vi "Pack for gRPC.vi"(8 "error in":errorcluster, 9 "configuration / results":enum16{"Configuration", "Results"}(ring), 10 "data value":variant, 11 "measurement customizations in":refnum<class "Measurement Plugin.lvclass">) -> (0 "error out":errorcluster, 2 "any":T1, 3 "measurement customizations out":refnum<class "Measurement Plugin.lvclass">)   [LabVIEW 2021, in "PWM Dimming.lvlib" / "Measurement Plugin.lvclass"]
uses:
  Measurement Plugin.lvclass
  Measurement Plugin.lvclass/Measurement Plugin.ctl
  Measurement Configuration.ctl
  PWM Dimming.lvlib
  Measurement Results.ctl
  a6012965-5700-4384-8228-972e71b6560c.vi
  2eca732d-dbaa-43bf-a7dd-ede2da65bc1b.vi
  <vilib>/Plug-In SDKs/Measurements/Measurement Plugin Service/Measurement Plugin Service.lvclass
  C:/Program Files/National Instruments/LabVIEW 2021/vi.lib/Plug-In SDKs/Measurements/Measurement Plugin Service/Measurement Plugin Service.lvclass
  <vilib>/gRPC/LabVIEW gRPC Library/Shared/Any.ctl
  <vilib>/gRPC/LabVIEW gRPC Library/grpc-lvsupport-release.lvlib
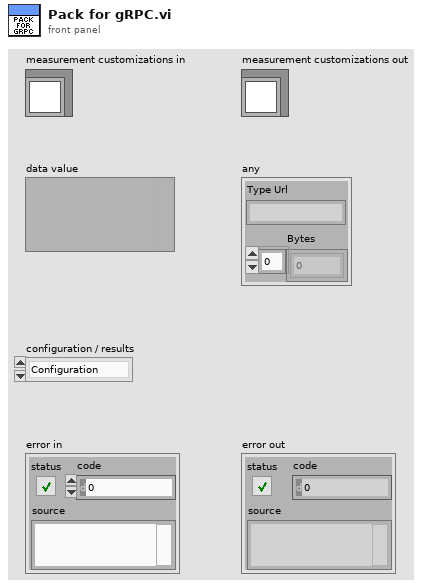
[diagram p1: front panel]
types:
  T1 = typedef "grpc-lvsupport-release.lvlib/Any.ctl" = cluster{"Type Url":string, "Bytes":u8[]}
  T2 = typedef "grpc-lvsupport-release.lvlib/grpcId.ctl" = u64
  T3 = typedef "PWM Dimming.lvlib/Measurement Configuration.ctl" = cluster{"DUT setup time":dbl, "Nominal output voltage":dbl, "Duty cycle single pulse/sweep pulse":bool, "PWM frequency":dbl, "Start duty cycle":dbl, "Stop duty cycle":dbl, "Number of sweep points":i32, "Duty cycle sweep type":string, "Duty cycle single point":dbl, "Number of pulse cycle":i32, "Source resource name":string, "Source sense":i32, "Source voltage level":dbl, "Source voltage level range":dbl, "Source transient response":i32, "Source voltage gain bandwidth":dbl, "Source voltage compensation frequency":dbl, "Source voltage pole-zero ratio":dbl, "Load resource name":string, "Load sense":i32, "Load pulse current level":dbl, "Load pulse bias current level":dbl, "Load sample rate":dbl, "Load voltage limit range":dbl, "Load transient response":i32, "Load current gain bandwidth":dbl, "Load current compensation frequency":dbl, "Load current pole-zero ratio":dbl, "Source current limit range":dbl, "AWG resource name":string, "AWG channel name":string, "AWG amplitude":dbl, "AWG dc offset":dbl, "Scope resource name":string, "Scope input channel name":string, "Scope sample rate":dbl, "Scope probe attenuation":dbl, "Scope vertical range":dbl, "Scope vertical coupling":enum32{"AC", "DC"}, "Load current level range":dbl, "AWG load impedence":dbl, "Measurement timeout":dbl, "AWG source trigger":string, "AWG measure trigger":string}
  T4 = typedef "PWM Dimming.lvlib/Measurement Results.ctl" = cluster{"Output voltages(SMU)":dbl[], "Output currents(SMU)":dbl[], "Input voltages(SMU)":dbl[], "SMU dt":dbl, "Scope dt":dbl, "PWM input voltage(scope amplitude)":dbl[], "Output duty cycle(%)":dbl[], "Input duty cycle(%)":dbl[]}
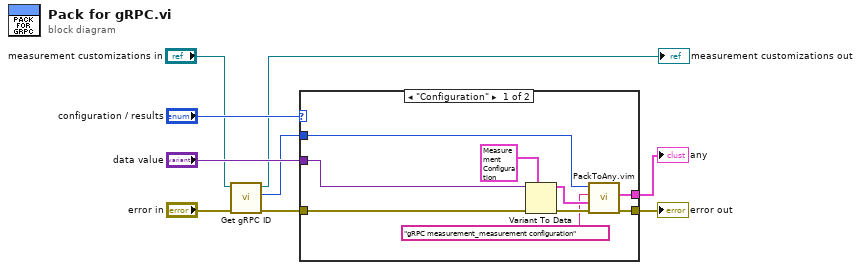
[diagram p0: block diagram]
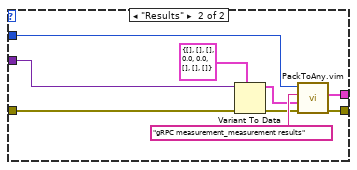
[diagram p2: hidden frame]
diagram:
  n1 = call <vilib>:"Get gRPC ID.vi"("error in"="error in", "measurement plugin service in"="measurement customizations in") -> ("error out"=w4:errorcluster, "gRPC ID"=w1:T2, "measurement plugin service out"=→"measurement customizations out":refnum<class "Measurement Plugin.lvclass">)  [unwired: 7 in]
  n2 = case shown="\"Configuration\"" "configuration / results" {
    tunnel: w4 -> [w18 w27]
    tunnel: "data value" -> [w17 w26]
    tunnel: w1 -> [w14 w22]
    tunnel: [w16 w24] -> w8
    tunnel: [w15 w23] -> w7
    frame "Configuration" {
      n3 = Variant To Data(error in=w18, type=T3 {"DUT setup time"=1.0, "Nominal output voltage"=3.3, "Duty cycle single pulse/sweep pulse"=TRUE, "PWM frequency"=25.0, "Start duty cycle"=0.9, "Stop duty cycle"=99.1, "Number of sweep points"=10, "Duty cycle sweep type"="Linear", "Duty cycle single point"=50.0, "Number of pulse cycle"=10, "Source resource name"="", "Source sense"=1009, "Source voltage level"=12.0, "Source voltage level range"=15.0, "Source transient response"=1042, "Source voltage gain bandwidth"=2000.0, "Source voltage compensation frequency"=3530.0, "Source voltage pole-zero ratio"=2.0, "Load resource name"="", "Load sense"=1009, "Load pulse current level"=-0.02, "Load pulse bias current level"=0.0, "Load sample rate"=1800000.0, "Load voltage limit range"=15.0, "Load transient response"=1038, "Load current gain bandwidth"=50000.0, "Load current compensation frequency"=250000.0, "Load current pole-zero ratio"=5.0, "Source current limit range"=0.1, "AWG resource name"="0", "AWG channel name"="", "AWG amplitude"=4.0, "AWG dc offset"=2.0, "Scope resource name"="", "Scope input channel name"="0", "Scope sample rate"=1800000.0, "Scope probe attenuation"=10.0, "Scope vertical range"=15.0, "Scope vertical coupling"=enum."DC", "Load current level range"=15.0, "AWG load impedence"=100000.0, "Measurement timeout"=10.0, "AWG source trigger"="PFI0", "AWG measure trigger"=""} ("measurement configuration"), Variant=w17) -> (data=w13:T3, error out=w12:errorcluster)
      n4 = call "PackToAny.vim"("error in"=w12, "Data To Pack"=w13, "Message Type"="gRPC measurement_measurement configuration", "gRPCid in"=w14) -> ("error out"=w16:errorcluster, "Any"=w15:T1)  [unwired: 5 in, 1 out]
    }
    frame "Results" {
      n5 = Variant To Data(error in=w27, type=T4 {"Output voltages(SMU)"=[], "Output currents(SMU)"=[], "Input voltages(SMU)"=[], "SMU dt"=0.0, "Scope dt"=0.0, "PWM input voltage(scope amplitude)"=[], "Output duty cycle(%)"=[], "Input duty cycle(%)"=[]} ("Measurement Results"), Variant=w26) -> (data=w20:T4, error out=w19:errorcluster)
      n6 = call "PackToAny.vim"("error in"=w19, "Data To Pack"=w20, "Message Type"="gRPC measurement_measurement results", "gRPCid in"=w22) -> ("error out"=w24:errorcluster, "Any"=w23:T1)  [unwired: 5 in, 1 out]
    }
  }
  "error out" <- w8
  "any" <- w7
